vi "Analysis.StartTime 1D to Throughput Graph.vi"(10 "Throughput Interval(Hrs)":dbl=1.0 caption="Interval(Hrs)", 11 "Start Times":timestamp[](array[timestamp])) -> (2 "Throughput table":string[][](table), 3 "Throughput Graph":cluster{"T":timestamp[], "Cnt":dbl[]}(graph) caption="Throughput Rate")   [LabVIEW 2024]
panel:
  out "Sum cnts":i32
  out "Record Cnt":i32
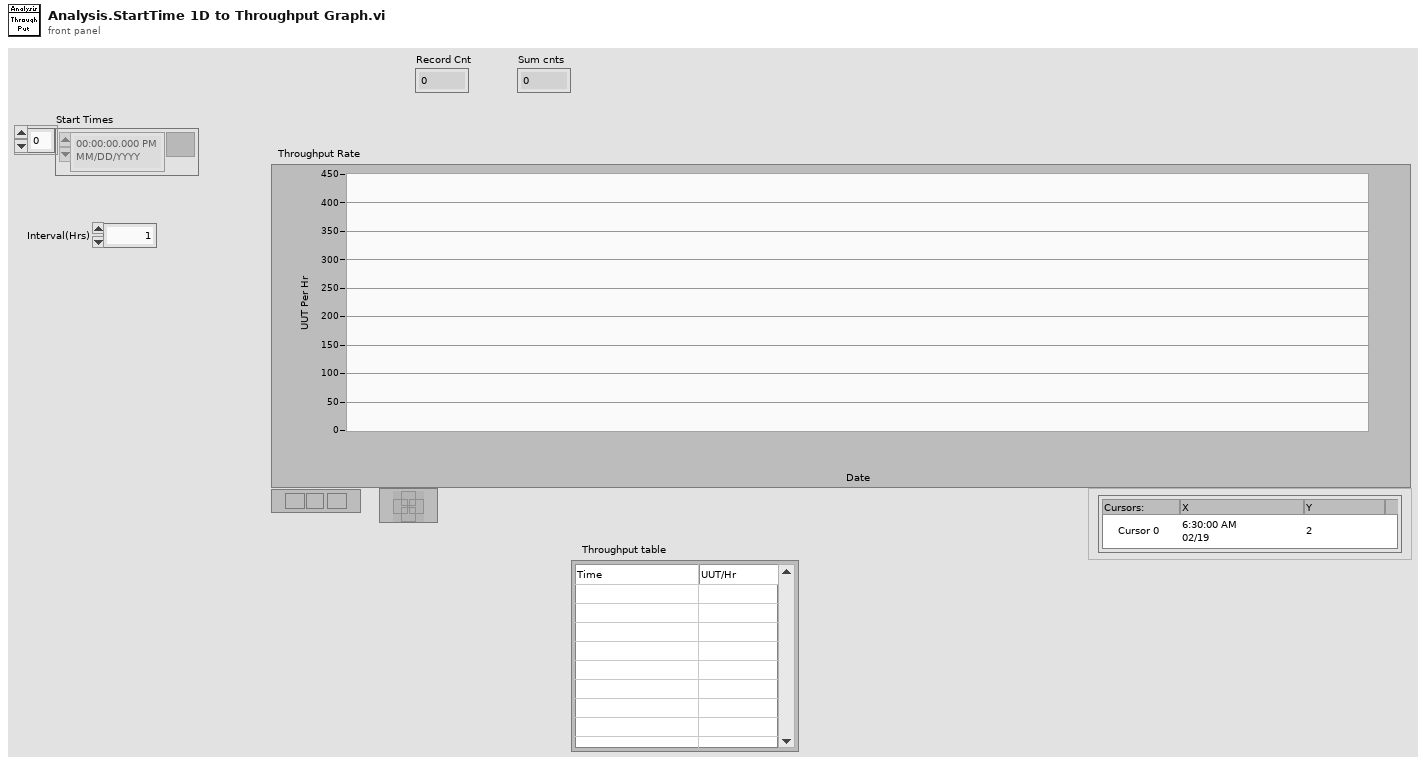
[diagram p1: front panel]
types:
  T1 = typedef "LVDateTimeRec.ctl" = cluster{"fractional second":dbl, "second":i32, "minute":i32, "hour":i32, "day of month":i32, "month":i32, "year":i32, "day of week":i32, "day of year":i32, "DST":i32}
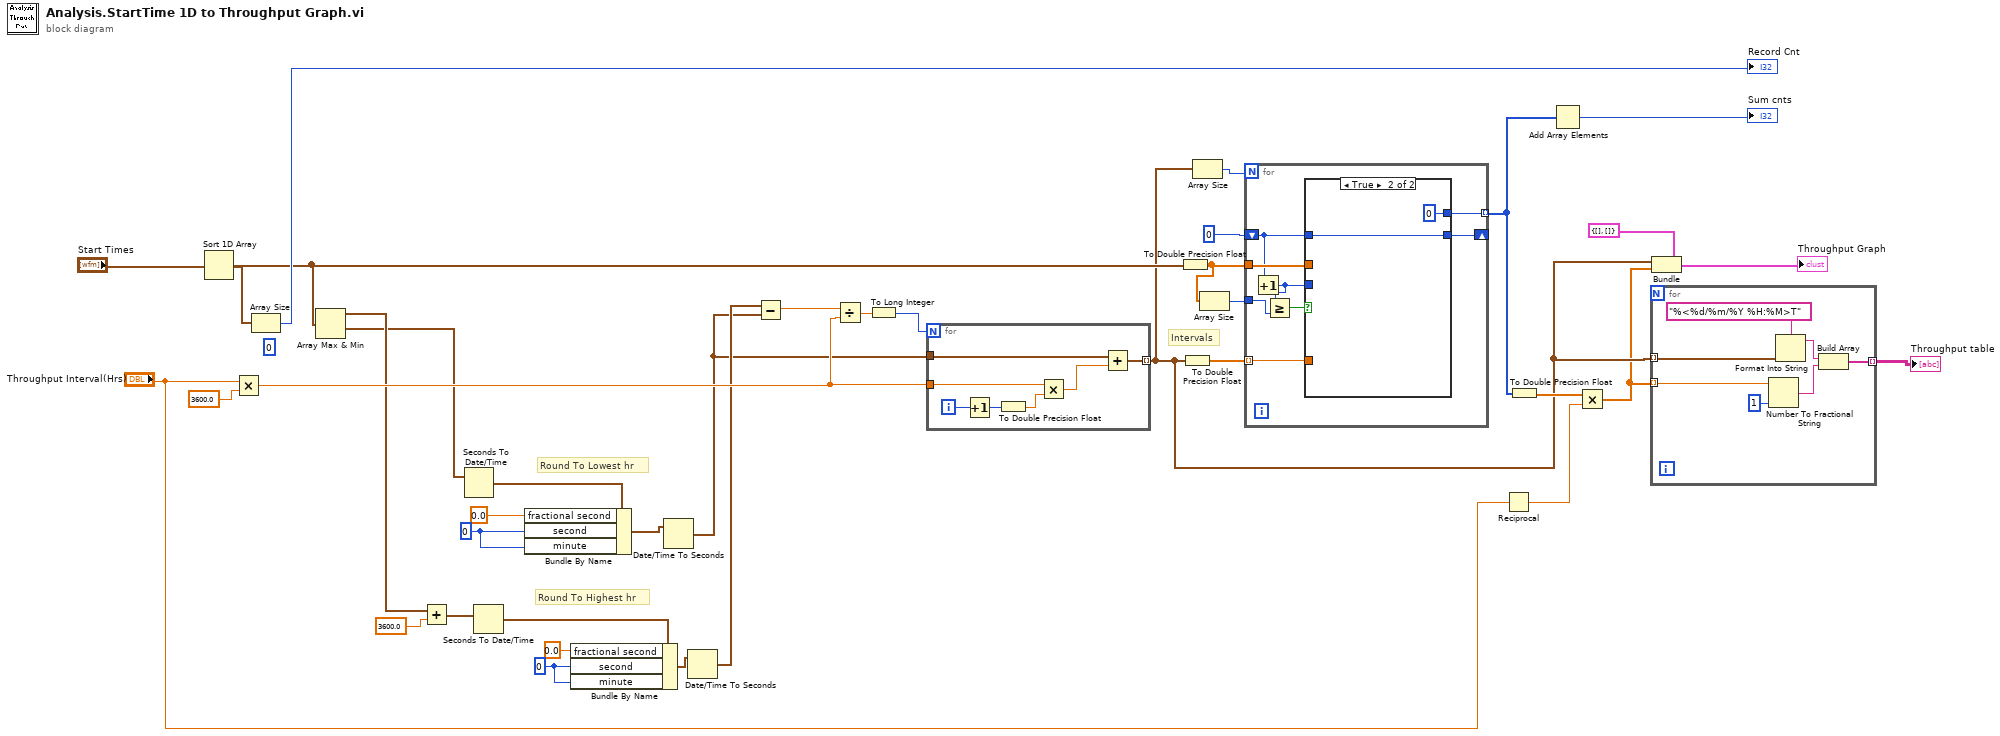
[diagram p0: block diagram]
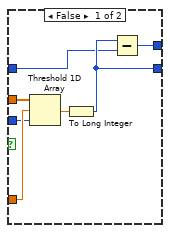
[diagram p2: hidden frame]
diagram:
  w22 = 0 ("second")
  w25 = 0 ("second")
  (unwired) 0
  # "Round To Highest hr"
  # "Round To Lowest hr"
  # "Intervals"
  n1 = Sort 1D Array(array="Start Times") -> (sorted array=w14:timestamp[])
  n2 = Multiply(x="Throughput Interval(Hrs)", y=3600.0) -> (x*y=w35:dbl)
  n3 = Array Size(array=w14) -> (size(s)=→"Record Cnt":i32)
  n4 = Array Max & Min(array=w14) -> (max value=w9:timestamp, min value=w8:timestamp)  [unwired: 2 out]
  n5 = Add(x=w9, y=3600.0) -> (x+y=w20:timestamp)
  n6 = Seconds To Date/Time(time stamp (now)=w8) -> (date time rec=w26:T1)  [unwired: 1 in]
  n7 = Seconds To Date/Time(time stamp (now)=w20) -> (date time rec=w21:T1)  [unwired: 1 in]
  n8 = Bundle By Name(cluster=w26, "fractional second"=0.0, "second"=w25, "minute"=w25) -> (w18:T1)
  n9 = Bundle By Name(cluster=w21, "fractional second"=0.0, "second"=w22, "minute"=w22) -> (w17:T1)
  n10 = Date/Time To Seconds(2:w18) -> (0:w6:timestamp)  [unwired: 1 in]
  n11 = Date/Time To Seconds(2:w17) -> (0:w7:timestamp)  [unwired: 1 in]
  n12 = Subtract(x=w7, y=w6) -> (x-y=w16:dbl)
  n13 = Divide(x=w16, y=w35) -> (x/y=w36:dbl)
  n14 = To Long Integer(number=w36) -> (32bit integer=w33:i32)
  n15 = for {
    N: w33 -> [_]
    tunnel: w6 -> [w42]
    tunnel: w35 -> [w43]
    tunnel: [w40] -> w5 mode=indexing
    i -> [w39]
    n16 = Increment(x=w39) -> (x+1=w38:i32)
    n17 = To Double Precision Float(number=w38) -> (double precision float=w44:dbl)
    n18 = Multiply(x=w43, y=w44) -> (x*y=w41:dbl)
    n19 = Add(x=w42, y=w41) -> (x+y=w40:timestamp)
  }
  n20 = To Double Precision Float(number=w14) -> (double precision float=w3:dbl[])
  n21 = To Double Precision Float(number=w5) -> (double precision float=w32:dbl[])
  n22 = Array Size(array=w5) -> (size(s)=w4:i32)
  n23 = Array Size(array=w3) -> (size(s)=w2:i32)
  n24 = for {
    N: w4 -> [_]
    tunnel: w3 -> [w52]
    tunnel: w32 -> [w51] mode=indexing
    shift-right: [w50] -> _
    shift-left: 0 -> [w48]
    tunnel: [w49] -> w13 mode=indexing
    tunnel: w2 -> [w46]
    n25 = Increment(x=w48) -> (x+1=w47:i32)
    n26 = Greater Or Equal?(x=w47, y=w46) -> (x >= y?=w45:bool)
    n27 = case shown="True" w45 {
      tunnel: w52 -> [w59 _]
      tunnel: w51 -> [w58 _]
      tunnel: [w57 w61] -> w50
      tunnel: [w56 0] -> w49
      tunnel: w48 -> [w55 w61]
      tunnel: w47 -> [w54 _]
      frame False {
        n28 = Threshold 1D Array(1:w54, 2:w58, 3:w59) -> (0:w53:dbl)
        n29 = To Long Integer(number=w53) -> (32bit integer=w57:i32)
        n30 = Subtract(x=w57, y=w55) -> (x-y=w56:i32)
      }
      frame True {
      }
    }
  }
  n31 = Reciprocal(x="Throughput Interval(Hrs)") -> (1/x=w12:dbl)
  n32 = To Double Precision Float(number=w13) -> (double precision float=w10:dbl[])
  n33 = Add Array Elements(numeric array=w13) -> (sum=→"Sum cnts":i32)
  n34 = Multiply(x=w10, y=w12) -> (x*y=w1:dbl[])
  n35 = for {
    tunnel: w5 -> [w65] mode=indexing
    tunnel: w1 -> [w68] mode=indexing
    tunnel: [w66] -> w27 mode=indexing
    n36 = Number To Fractional String(number=w68, precision (6)=i16 1) -> (F-format string=w67:string)  [unwired: 2 in]
    n37 = Format Into String(format string="%<%d/%m/%Y %H:%M>T", w65) -> (resulting string=w63:string)  [unwired: 2 in, 1 out]
    n38 = Build Array(w63, w67) -> (w66:string[])
  }
  "Throughput table" <- w27
  n39 = Bundle(cluster=cluster{"T":timestamp[], "Cnt":dbl[]} {"T"=[], "Cnt"=[]}, "T"=w5, "Cnt"=w1) -> (→"Throughput Graph":cluster{"T":timestamp[], "Cnt":dbl[]})
